vi "rethinkdb_msg_handshake_initial.vi"(8 "error in (no error)":errorcluster, 10 "password":string, 11 "user":string) -> (0 "error out":errorcluster, 1 "client_first_message":string, 2 "dup password":string, 3 "initial_message":string, 4 "protocol_version":i32)   [LabVIEW 2017]
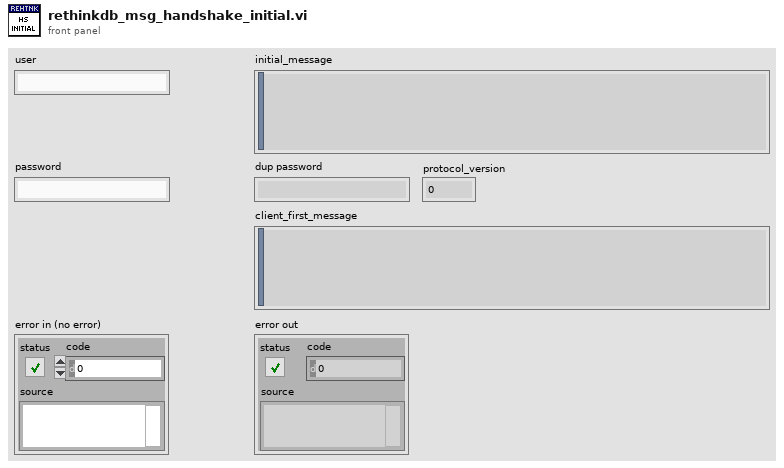
[diagram p1: front panel]
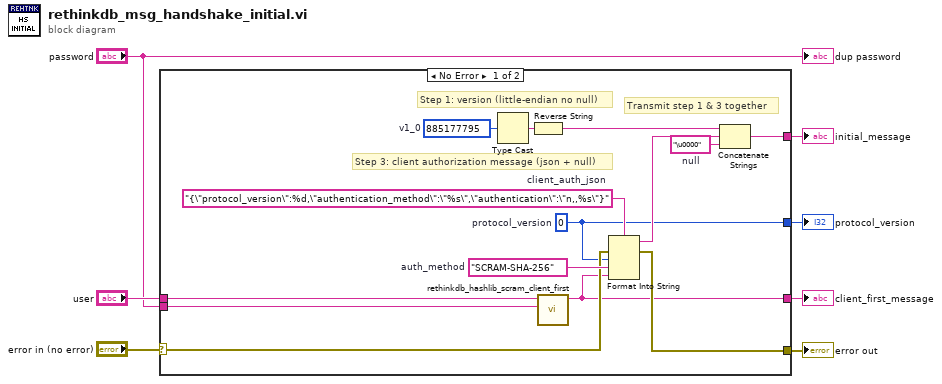
[diagram p0: block diagram]
diagram:
  n1 = case shown="No Error" "error in (no error)" {
    selector: "error in (no error)" -> [w12 w22]
    tunnel: "password" -> [w9 _]
    tunnel: "user" -> [w10 _]
    tunnel: [w14 w22] -> w5
    tunnel: [w19 _] -> w4
    tunnel: [w11 _] -> w3
    tunnel: [w8 _] -> w1
    frame No Error {
      w15 = "SCRAM-SHA-256"  # auth_method
      w8 = 0  # protocol_version
      w16 = "{\"protocol_version\":%d,\"authentication_method\":\"%s\",\"authentication\":\"n,,%s\"}"  # client_auth_json
      w17 = "\u0000"  # null
      w21 = 885177795  # v1_0
      # "Step 3: client authorization message (json + null)"
      # "Transmit step 1 & 3 together"
      # "Step 1: version (little-endian no null)"
      n2 = Type Cast(x=w21) -> (*(type *) &x=w20:string)  [unwired: 1 in]
      n3 = Reverse String(1:w20) -> (0:w18:string)
      n4 = call "rethinkdb_hashlib_scram_client_first.vi"("password"=w9, "user"=w10) -> ("client_first_message"=w11:string)  [unwired: 9 in]
      n5 = Format Into String(format string=w16, error in=w12, w8, w15, w11) -> (resulting string=w13:string, error out=w14:errorcluster)  [unwired: 1 in]
      n6 = Concatenate Strings(w18, w13, w17) -> (w19:string)
    }
    frame Error {
    }
  }
  "error out" <- w5
  "initial_message" <- w4
  "client_first_message" <- w3
  "protocol_version" <- w1
  "dup password" <- "password"
